vi "meetCriteria.vi"(8 "error in (no error)":errorcluster, 10 "Persons In":refnum<class "Person.lvclass">[](array[class]), 11 "CriteriaFemale in":refnum<class "CriteriaFemale.lvclass">) -> (0 "error out":errorcluster, 2 "Persons Out":refnum<class "Person.lvclass">[](array[class]), 3 "CriteriaFemale out":refnum<class "CriteriaFemale.lvclass">)   [LabVIEW 2018, in "CriteriaFemale.lvclass"]
uses:
  CriteriaFemale.lvclass
  Person Class/Person.lvclass
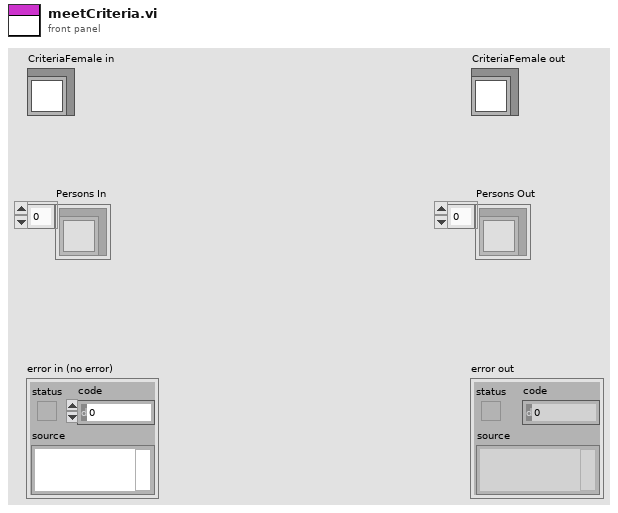
[diagram p1: front panel]
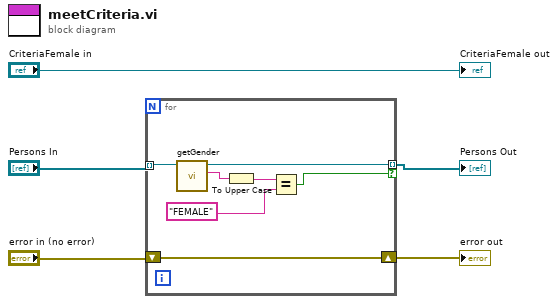
[diagram p0: block diagram]
diagram:
  n1 = for {
    shift-right: [w12] -> w4
    shift-left: "error in (no error)" -> [w12]
    tunnel: "Persons In" -> [w11] mode=indexing
    tunnel: [w7] -> w1 mode=indexing if=w6
    n2 = call-dynamic "getGender.vi"("Person in"=w11) -> ("gender"=w10:string, "Person out"=w7:refnum<class "Person.lvclass">)  [unwired: 8 in, 1 out]
    n3 = To Upper Case(1:w10) -> (0:w9:string)
    n4 = Equal?(x=w9, y="FEMALE") -> (x = y?=w6:bool)
  }
  "error out" <- w4
  "Persons Out" <- w1
  "CriteriaFemale out" <- "CriteriaFemale in"
